vi "c ctre phoenixpro Set Update Frequency.vi"(5 "timeoutSeconds":dbl, 6 "frequencyHz":dbl, 7 "spn":u16, 8 "error in (no error)":errorcluster, 9 "deviceHash":u32, 10 "network":string, 11 "context":u32(ring) items=["ContextAPI", "ContextDiagServer"]) -> (0 "error out":errorcluster, 3 "function return":i32)   [LabVIEW 2020, in "CTRE_PhoenixTools.lvlib"]
doc: "CTREXPORT int c_ctre_phoenixpro_SetUpdateFrequency(Context context, const char *network, uint32_t deviceHash, uint16_t spn, double frequencyHz, double timeoutSeconds);"
uses:
  <userlib>/CTRE_PhoenixTools/CTRE_PhoenixTools.lvlib
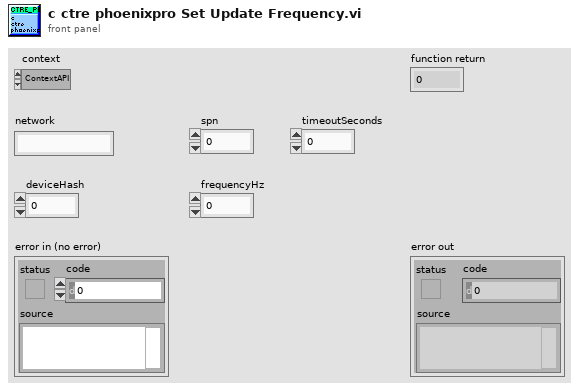
[diagram p1: front panel]
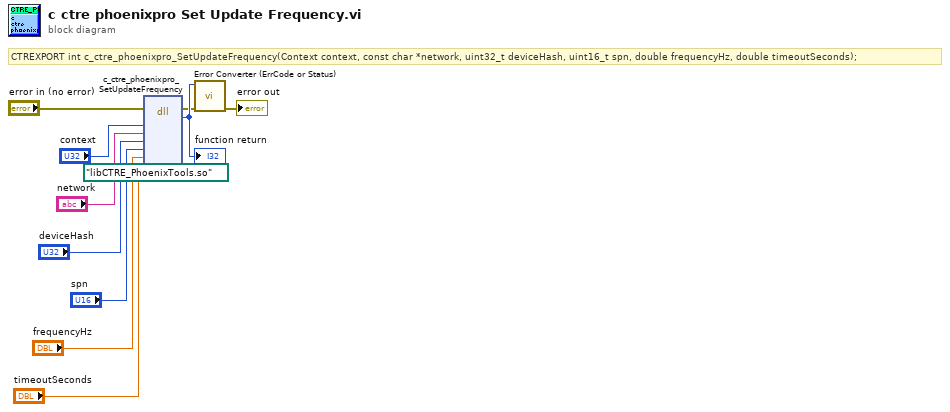
[diagram p0: block diagram]
diagram:
  # "CTREXPORT int c_ctre_phoenixpro_SetUpdateFrequency(Context context, const char *network, uint32_t deviceHash, uint16_t spn, double frequencyHz, double timeoutSeconds);"
  n1 = dll-call lib="?" fn="c_ctre_phoenixpro_SetUpdateFrequency"(path in=path "libCTRE_PhoenixTools.so", error in="error in (no error)", "context"="context", "network"="network", "deviceHash"="deviceHash", "spn"="spn", "frequencyHz"="frequencyHz", "timeoutSeconds"="timeoutSeconds") -> (error out=w3:errorcluster, w11:i32)  [unwired: 7 in, 1 out]
  "function return" <- w11
  n2 = call <userlib>:"Error Converter (ErrCode or Status).vi"("error in (no error)"=w3, "error code"=w11) -> ("error out"=→"error out":errorcluster)  [unwired: 9 in]
